vi "Addressing_add_1_afterLast1.vi"(8 "error in (no error)":errorcluster, 11 "VALUE":u32=121 format="%08b") -> (0 "error out":errorcluster, 2 "Last value":bool, 3 "Value + next 1":u32 format="%08b")   [LabVIEW 2014, in "Driver_interaction.lvlib" / "Dali_usb_tridonics.lvclass"]
doc: "Add a \"1\" after that the last \"1\".\nFor example:\n1001 0000 -> 1001 1000"
uses:
  Dali_usb_tridonics.lvclass
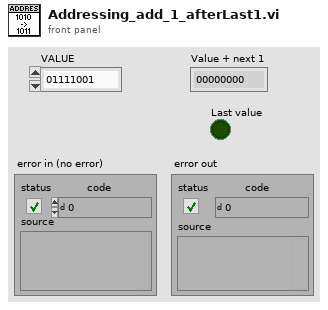
[diagram p1: front panel]
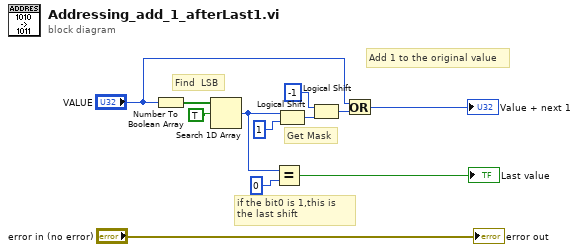
[diagram p0: block diagram]
diagram:
  # "Add 1 to the original value"
  # "if the bit0 is 1,this is the last shift"
  # "Get Mask"
  # "Find  LSB"
  n1 = Number To Boolean Array(number="VALUE") -> (Boolean array=w9:bool[])
  n2 = Search 1D Array(1D array=w9, element=TRUE) -> (index of element=w4:i32)  [unwired: 1 in]
  n3 = Equal?(x=w4, y=0) -> (x = y?=→"Last value":bool)
  n4 = Logical Shift(y=w4, x=u32 1) -> (x << y=w5:u32)
  n5 = Logical Shift(y=i16 -1, x=w5) -> (x << y=w10:u32)
  n6 = Or(x="VALUE", y=w10) -> (x .or. y?=→"Value + next 1":u32)
  "error out" <- "error in (no error)"
